vi "Read Pretty Print.vi"(8 "error in (no error)":errorcluster, 11 "Serializer.JDP-JSON in":refnum<class "Serializer.JDP-JSON.lvclass">) -> (0 "error out":errorcluster, 2 "Pretty Print":bool=TRUE, 3 "Serializer.JDP-JSON out":refnum<class "Serializer.JDP-JSON.lvclass">)   [LabVIEW 2019, in "OpenSerializer.JDP-JSON.lvlib" / "Serializer.JDP-JSON.lvclass"]
uses:
  Serializer.JDP-JSON.lvclass
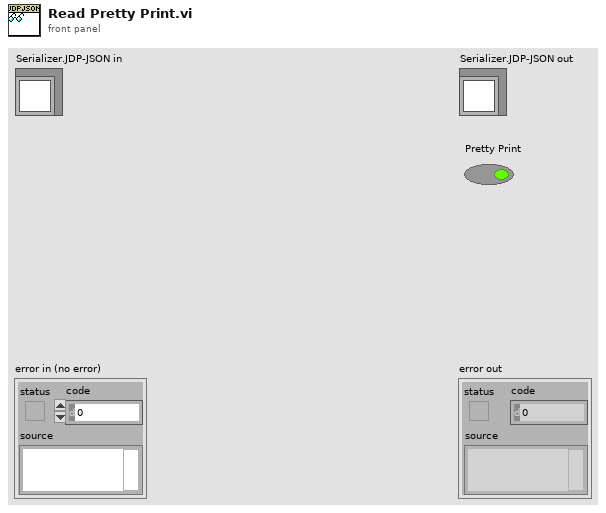
[diagram p1: front panel]
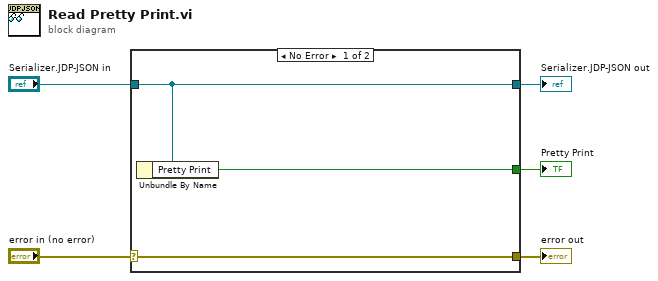
[diagram p0: block diagram]
diagram:
  n1 = case shown="No Error" "error in (no error)" {
    selector: "error in (no error)" -> [w8 w9]
    tunnel: [w8 w9] -> w4
    tunnel: [w7 w10] -> w2
    tunnel: "Serializer.JDP-JSON in" -> [w7 w10]
    tunnel: [w6 _] -> w1
    frame No Error {
      n2 = Unbundle By Name(w7) -> ("Pretty Print"=w6:bool)
    }
    frame Error {
    }
  }
  "error out" <- w4
  "Serializer.JDP-JSON out" <- w2
  "Pretty Print" <- w1
